vi "TestSbig.vi"() -> ()   [LabVIEW 2009]
panel:
  in  "Window":bool
  in  "Time":u32
  in  "stop":bool
  out "Graphe intensity":i32[][](graph)
  in  "SBIG Name":string
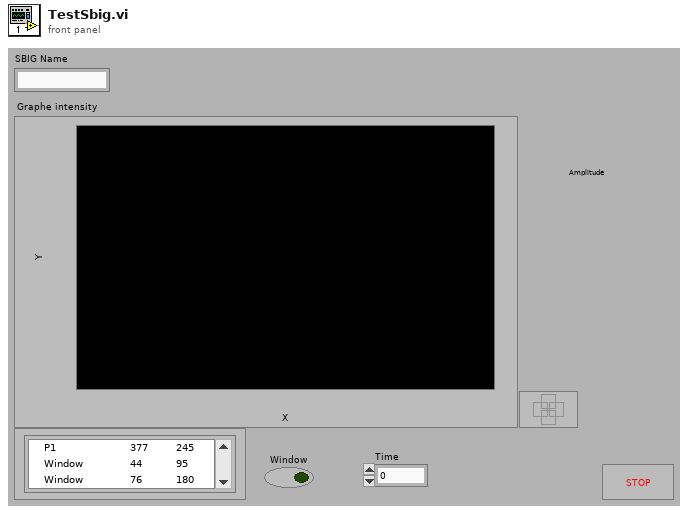
[diagram p1: front panel]
types:
  T1 = cluster{"X0":u16, "Y0":u16, "DX":u16, "DY":u16, "on/off":bool}
  T2 = typedef "LVCursorListTypeDef.ctl" = cluster{"Name":string, "Color":u32, "Style":u8, "Point Style":u8, "Name Visible":bool, "Allow Drag":bool, "Cursor Mode":u32, "Plot":i32, "Index":i32, "Position":cluster{"X":dbl, "Y":dbl}, "X Scale":u32, "Y Scale":u32, "Watch Plots":i32[], "Watch All Plots":bool, "Plot Area":i32, "Label Offset":cluster{"X":dbl, "Y":dbl}}[]
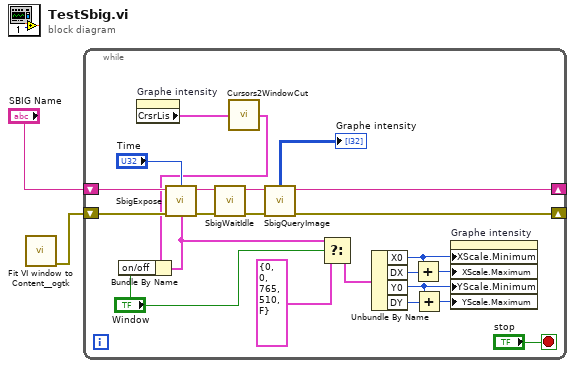
[diagram p0: block diagram]
diagram:
  n1 = call <userlib>:"Fit VI window to Content__ogtk.vi"() -> ("error out"=w1:errorcluster)  [unwired: 3 in, 4 out]
  n2 = while {
    shift-right: [w22] -> _
    shift-left: w1 -> [w23]
    shift-right: [w20] -> _
    shift-left: "SBIG Name" -> [w24]
    stop <- "stop" stop-if-true
    n3 = property on="Graphe intensity" class="IntGraph (strict)"() -> ("CrsrLis"=w6:T2)  [unwired: 2 in, 2 out]
    n4 = call "Cursors2WindowCut.vi"("Cursor List"=w6) -> ("Window"=w5:T1)
    n5 = Bundle By Name(cluster=w5, "on/off"="Window") -> (w3:T1)
    n6 = call "SbigExpose.vi"("Time"="Time", "Sbig"=w24, "Window"=w3, "error in (no error)"=w23) -> ("Sbig out"=w18:string, "error out"=w16:errorcluster)  [unwired: 4 out]
    n7 = call "SbigWaitIdle.vi"("error in (no error)"=w16, "Sbig Name"=w18) -> ("error out"=w15:errorcluster, "Sbig Name Out"=w17:string)  [unwired: 8 out]
    n8 = call "SbigQueryImage.vi"("Sbig"=w17, "error in (no error)"=w15) -> ("Sbig out"=w20:string, "Image"=→"Graphe intensity":i32[][], "error out"=w22:errorcluster)  [unwired: 5 out]
    n9 = Select(t=w3, s="Window", f=T1 {"X0"=0, "Y0"=0, "DX"=765, "DY"=510, "on/off"=FALSE} ("Window")) -> (s? t:f=w7:T1)
    n10 = Unbundle By Name(w7) -> ("X0"=w14:u16, "DX"=w13:u16, "Y0"=w10:u16, "DY"=w9:u16)
    n11 = Add(x=w14, y=w13) -> (x+y=w12:u16)
    n12 = Add(x=w10, y=w9) -> (x+y=w11:u16)
    n13 = property on="Graphe intensity" class="IntGraph (strict)"("XScale.Minimum"=w14, "XScale.Maximum"=w12, "YScale.Minimum"=w10, "YScale.Maximum"=w11) -> ()  [unwired: 2 in, 2 out]
  }
